vi "VI Tree.vi"   [LabVIEW 2015, in "Template - Counter.lvlib"]
doc: "This is the instrument driver for the <INSTRUMENT NAME>. The VI Tree displays all the user-callable VIs of the instrument driver in an organized table."
uses:
  <instrlib>/_Template - Counter/Template - Counter.lvlib
  <instrlib>/_Template - Counter/Public/Configure/Configure Measurement (Frequency).vi
panel:
  # "(c) 2014 <Enter Company Name Here>.  ALL RIGHTS RESERVED."
  # "SEE DIAGRAM\nFOR VI TREE."
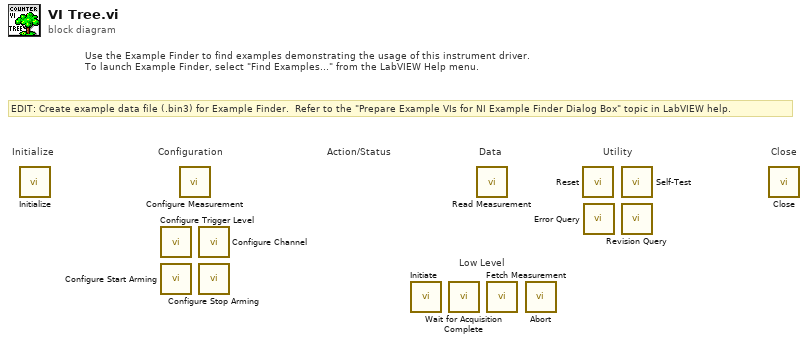
[diagram p0: block diagram]
diagram:
  # "Low Level"
  # "EDIT: Create example data file (.bin3) for Example Finder.  Refer to the \"Prepare Example VIs for NI Example Finder Dialog Box\" topic in LabVIEW help."
  # "Use the Example Finder to find examples demonstrating the usage of this instrument driver.\nTo launch Example Finder, select \"Find Examples...\" from the LabVIEW Help menu."
  # "Configuration"
  # "Utility"
  # "Data"
  # "Action/Status"
  # "Close"
  # "Initialize"
  n1 = call <instrlib>:"Initialize.vi"() -> ()  [unwired: 10 in, 2 out]
  n2 = call <instrlib>:"Configure Trigger Level.vi"() -> ()  [unwired: 10 in, 2 out]
  n3 = call <instrlib>:"Configure Start Arming.vi"() -> ()  [unwired: 10 in, 2 out]
  n4 = call-poly <instrlib>:"Configure Measurement.vi"() -> ()  [unwired: 10 in, 2 out]
  n5 = call <instrlib>:"Configure Channel.vi"() -> ()  [unwired: 10 in, 2 out]
  n6 = call <instrlib>:"Configure Stop Arming.vi"() -> ()  [unwired: 10 in, 2 out]
  n7 = call <instrlib>:"Initiate.vi"() -> ()  [unwired: 10 in, 2 out]
  n8 = call <instrlib>:"Wait for Acquisition Complete.vi"() -> ()  [unwired: 10 in, 2 out]
  n9 = call <instrlib>:"Read Measurement.vi"() -> ()  [unwired: 9 in, 3 out]
  n10 = call <instrlib>:"Fetch Measurement.vi"() -> ()  [unwired: 9 in, 3 out]
  n11 = call <instrlib>:"Abort.vi"() -> ()  [unwired: 10 in, 2 out]
  n12 = call <instrlib>:"Reset.vi"() -> ()  [unwired: 10 in, 2 out]
  n13 = call <instrlib>:"Error Query.vi"() -> ()  [unwired: 8 in, 4 out]
  n14 = call <instrlib>:"Self-Test.vi"() -> ()  [unwired: 8 in, 4 out]
  n15 = call <instrlib>:"Revision Query.vi"() -> ()  [unwired: 8 in, 4 out]
  n16 = call <instrlib>:"Close.vi"() -> ()  [unwired: 11 in, 1 out]
